vi "FDD Self TRAINING Polynomial FIT Ver07.vi"(4 "Remove Coefficient\nif makes < X% Change in SSE":dbl=1.0, 5 "DO Backward Elimination\nto REDUCE # Coefficients?":bool, 7 "No Header Labels?":bool, 8 "Select Polynomial Order":u16(ring) items=["1st ORDER", "2nd ORDER", "3rd Order"], 9 "Dependent Variable\nCOLUMN INDICES":i32[](array[numeric])=[5, 6, 8, 9, 12, 22, 39, 40, 46, 47, 48, 49, 54, 58, 64, 65, 69, 77, 81, 82, 87, 90, 92, 93, 105, 134, 135, 185, 188, 191, 192, 194, 206, 207, 208, 209, 210, 211, 219, 220, 222, 223, 225, 226, 227, 228, 229, 230, 231, 232, 233, 234, 237, 240, 241, 245, 246, 252, 254, 255, 256, 258, 260, 267, 268, 269], 10 "THREE Independent Variables\nCOLUMN INDICES":i32[](array[numeric])=[182, 83, 195]) -> (0 "# of Points (ROWS)":i32, 1 "Dependent VARIABLE(S) Numeric Data Array":dbl[][](array[numeric]), 2 "Independent VARIABLES, x1, x2, x3 -  Numeric Data Array":dbl[][](array[numeric]), 3 "Reduced Model(s) Coefficients with MSE, DOF(N-m), Student T-Value, and Model 95% CI (on Mean) in last four columns of the row":string[][](array[string]), 11 "RAW Data Array - STRING":string[][](array[string])=[["Hughie", "Dewey", "Louie", "Daffy", "Daisy"], ["1", "11", "4587", "4756", "12"], ["4", "55", "46", "5458", "45"], ["2", "22", "4789", "4445", "44"], ["7", "77", "258", "7595", "78"], ["9", "22", "1125", "147", "44545"], ["12", "33", "567", "233", "44"], ["32", "88", "413", "546", "895"], ["23", "65", "789", "7778", "458"], ["67", "99", "599", "6754", "478"], ["2111", "345", "678", "4399", "155"], ["199", "34", "555", "3987", "225"], ["37", "145", "258", "458", "3655"], ["876", "74", "635", "1258", "479"], ["45", "69", "158", "635", "258"], ["23", "125", "365", "489", "895"], ["11", "48", "428", "569", "965"], ["78", "79", "123", "45", "995"], ["65", "225", "754", "478", "788"], ["11", "48", "982", "569", "774"], ["97", "49", "4289", "483", "258"], ["38", "698", "1587", "147", "88"]])   [LabVIEW 2017]
uses:
  Control 1.ctl
  <vilib>/Analysis/6fits.llb/Curve Fitting Criteria.ctl
  <vilib>/Analysis/6fits.llb/General Linear Fit Algorithm.ctl
  <vilib>/Analysis/baseanly.llb/Mean (DBL).vi
  <vilib>/Utility/file.llb/Read Delimited Spreadsheet (string).vi
  <vilib>/Utility/file.llb/Write Delimited Spreadsheet (string).vi
  <vilib>/gmath/statdist.llb/st_Percentiles (scalar).vi
  <vilib>/Analysis/NI_AALPro.lvlib
  <vilib>/Analysis/NI_AALBase.lvlib
  <vilib>/gmath/NI_Gmath.lvlib
panel:
  out "Full Model # of Coef.":i32
  out "Current Input FILE":string
  out "STOPPED 2":bool
  out "STOPPED":bool
  out "General Linear FIT error out":errorcluster
  in  "Tab Control":T1(tab)
  in  "SAVE?":bool
  in  "Saved Coefficient File":path=path "C:/TEMP/Coef_JUNK_Goodman_SHORT_COOL_NFSS_ALL_161207.txt"
  in  "Process\nData ??":bool
  in  "Input File":path=path "C:/Vance/FDD Split System Project/FDD_LOW-HIGH_EfficiencyHP_Testing/Goodman 14SEER Single-Speed HP LOW EFF UNIT TESTS 2015-16/SHORT LINESET DATA/Test DATA/BINS_Goodman_SHORT_COOL_NFSS_ALL_161207.txt"
  out "Save Coeff error out":errorcluster
  out "RAW Data COLUMN HEADER LABELS":string[](array[string])
  in  "Array of Calculated Variables (stuck in columns at end of Data Array String)":T3(array[cluster])=[{"Test Function"=7, "USE CONST."=FALSE, "CONSTANT"=1.0, "DATA COLUMNS"=[56.0, 60.0], "NEW HEADER LABEL"="ODAir_Exit_TempF"}, {"Test Function"=8, "USE CONST."=FALSE, "CONSTANT"=1.0, "DATA COLUMNS"=[266.0, 195.0], "NEW HEADER LABEL"="ODAir_DT(F)"}, {"Test Function"=8, "USE CONST."=FALSE, "CONSTANT"=1.0, "DATA COLUMNS"=[82.0, 105.0], "NEW HEADER LABEL"="LiqLine_DP(psid)"}]
  out "RAW & Calculated Data COLUMN HEADER LABELS":string[](array[string])
  in  "PAUSE to Select Independent \nand Dependent Data COLUMNS":bool
  out "RAW & CALCULATED Data Array - STRING":string[][](array[string])=[["Hughie", "Dewey", "Louie", "Daffy", "Daisy"], ["1", "11", "4587", "4756", "12"], ["4", "55", "46", "5458", "45"], ["2", "22", "4789", "4445", "44"], ["7", "77", "258", "7595", "78"], ["9", "22", "1125", "147", "44545"], ["12", "33", "567", "233", "44"], ["32", "88", "413", "546", "895"], ["23", "65", "789", "7778", "458"], ["67", "99", "599", "6754", "478"], ["2111", "345", "678", "4399", "155"], ["199", "34", "555", "3987", "225"], ["37", "145", "258", "458", "3655"], ["876", "74", "635", "1258", "479"], ["45", "69", "158", "635", "258"], ["23", "125", "365", "489", "895"], ["11", "48", "428", "569", "965"], ["78", "79", "123", "45", "995"], ["65", "225", "754", "478", "788"], ["11", "48", "982", "569", "774"], ["97", "49", "4289", "483", "258"], ["38", "698", "1587", "147", "88"]]
  out "Selected CASE":i32
  out "H Matrix":dbl[][](array[numeric])
  out "FULL Dataset Correlation Coefficients  and MSE in last column of the row (a0, a1, a2, ......., MSE)":dbl[][](array[numeric]) format="%_8e"
  in  "Outlier IQR Multiplier (k)":dbl=2.2
  out "Residuals for all Dependent Variables (Value Minus Fit Value)":dbl[][](array[numeric]) format="%_8e"
  out "STATS Columns for each Dependent Variable's Residuals":dbl[][](array[numeric]) format="%_4p"
  out "% of Data = OUTLIER":dbl format="%_3f"
  out "# OUTLIERS":i32
  out "# Datapoints in File":i32
  out "Residual's Variable NAME 2":string
  out "Line Numbers w/ OUTLIERS":bool[](array[boolean])
  out "Outlier Identified (Row is Line #, Column is Variable #)":bool[][](array[boolean])
  out "Column w/ OUTLIER??":cluster{"Variable LABEL NAME":string, bool}[](array[cluster])
  out "Residual's Histogram Graph":T4(graph)
  in  "Histogram\nSelected COL":i32
  out "Residual Value vs Line # XY Graph":cluster{"Y":dbl[], "Y":dbl[]}[](graph)
  out "Skewness":dbl
  out "Kurtosis":dbl
  out "Residual's Variable NAME":string
  out "STATISTICS - Array 3":T5(array[cluster])
  out "STATISTICS - Array 2":T5(array[cluster])
  out "STATISTICS - Array":T5(array[cluster])
  out "TOSS OUT Coefficients indicated by RED LED's":bool[][](array[boolean])
  out "Reduced Model's H Matrix":dbl[][](array[numeric])
  out "F-Test----SSE Reduced Model(s) Divided by SSE Full Model = SSE Ratio":dbl[][](array[numeric]) format="%.3p"
  out "SSE Full Model(s)":dbl[](array[numeric])
  out "SSE Ratio Must Be < THIS \nto Throw Out the Coeff.":dbl format="%#_6p"
  out "ERROR CODE":i32
  out "Dependent \nVariable INDEX":i32
  in  "10 sec Pause\nSTEP to Debug?":bool
  out "Fitted Coefficients MATRIX \nAssociated with H-Matrix w/ MSE at END":dbl[](array[numeric])
  out "Dependent Variable MATRIX \nAssociated with H-Matrix":dbl[](array[numeric])
  out "H-Matrix AFTER ZERO Value COLS ADDED":dbl[][](array[numeric]) format="%_9e"
  out "Coefficients with MSE in last Column-NUMERIC ARRAY":dbl[][](array[numeric]) format="%_9e"
  out "Reduced Model \n# of Coefficients":i32
  out "#COLS":i32
  # "Multivariate Polynomial FIT with 3 Independent Variables"
  # "y = a0*y0 + a1*y1 + .....+ai*yi  \nwhere i =0 to 19.\ny0=1;\ny1=x1;\ny2=x2;              1st Order\ny3=x3;\n--------------\ny4=x1*x2;\ny5=x1*x3;\ny6=x2*x3;\ny7=x1**2;        2nd Order\ny8=x2**2;\ny9=x3**2;\n----------------\ny10=x1*x2*x3;\ny11=x1*x2**2;\ny12=x1*x3**2;\ny13=x2*x3**2;\ny14=x1**2*x2;  3rd Order\ny15=x1**2*x3;\ny16=x2**2*x3;\ny17=x1**3;\ny18=x2**3;\ny19=x3**3;"
  # "Needs to be a Tab Delimited Text file \nwith data in columns."
  # "Max\nMin\nMedian\nQuartile 1 (25%)\nQuartile 3 (75%)\nInterQuartileRange (3-1)\nOutlier LowerBound\nOutlier UpperBound"
  # "LowerBound = Q1 - k * IQR\nUpperBound = Q3 + k * IQR"
  # "Assumes Residuals are normally distributed about zero."
  # "A negative value of skewness indicates \nthat the left side of the probability density \nfunction is longer than the right side. A \npositive value of skewness indicates that \nthe right side of the probability density \nfunction is longer than the left side."
  # "A normal distribution has a kurtosis value \nof 3. A kurtosis value of less than 3 indicates \na flatter distribution than normal. A kurtosis \nvalue of greater than 3 indicates a sharper \ndistribution than normal."
  # "For Example:\n(0,0) is the SSE Ratio after removing a0 from Model 0\n(1,2) is the SSE Ratio after removing a2 from Model 2"
  # "If you have only one Independent Variable,\nthen you will have only ONE row of SSE ratio."
  # "Each COL is replaced by 0's in sequence to remove the coefficent from the fit.  \nFinal ARRAY will show all 0's in the last COL."
  # "Degrees of Freedom\n= DOF = #Points-#Coef = N-m"
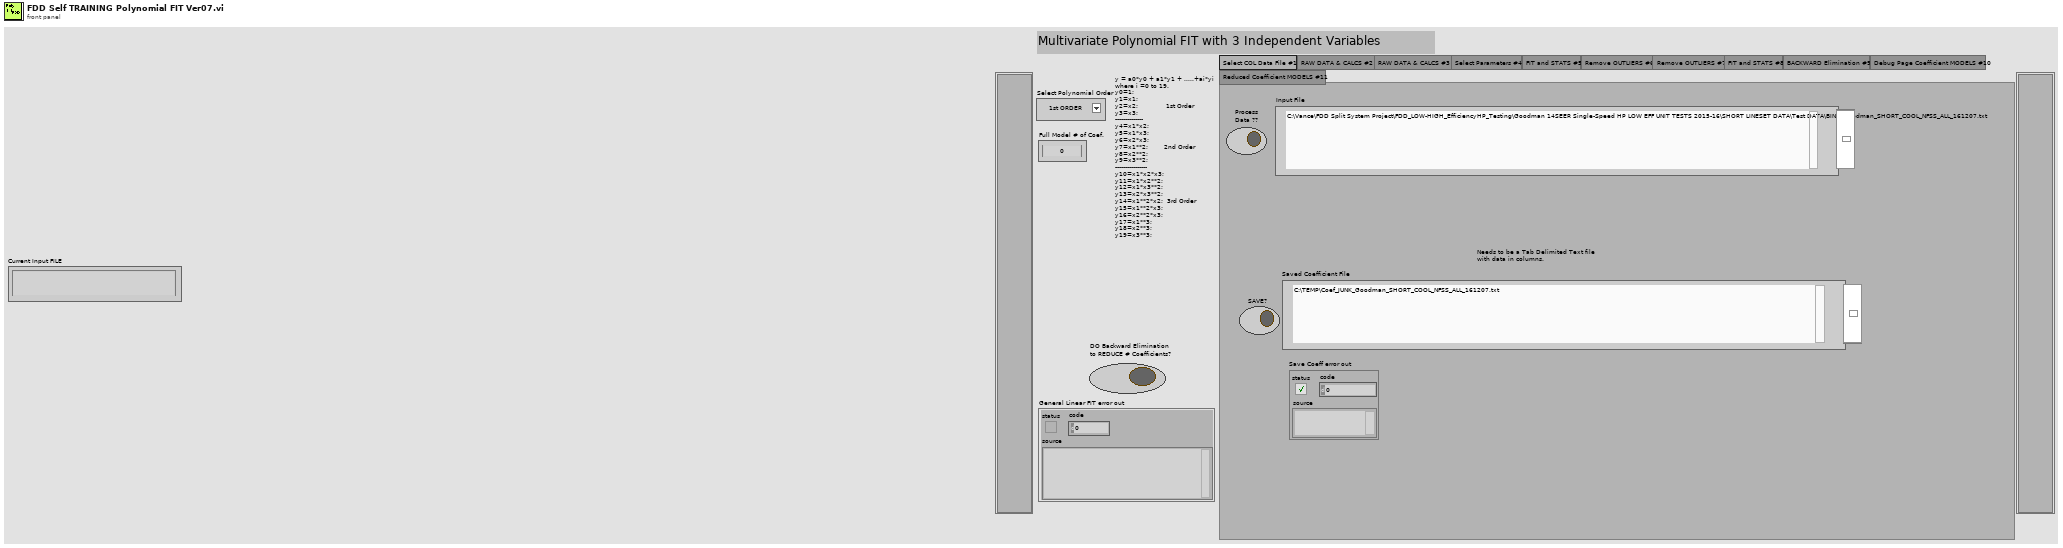
[diagram p1: front panel]
types:
  T1 = enum32{"Select COL Data File #1", "RAW DATA & CALCS #2", "RAW DATA & CALCS #3", "Select Parameters #4", "FIT and STATS #5", "Remove OUTLIERS #6", "Remove OUTLIERS #7", "FIT and STATS #8", "BACKWARD Elimination #9", "Debug Page Coefficient MODELS #10", "Reduced Coefficient MODELS #11"}
  T2 = typedef "Control 1.ctl" = i32
  T3 = cluster{"Test Function":T2, "USE CONST.":bool, "CONSTANT":dbl, "DATA COLUMNS":dbl[], "NEW HEADER LABEL":string}[]
  T4 = cluster{"X Values":dbl[], "Histogram: h(x)":i32[]}
  T5 = cluster{"Header":string, "Mean":dbl, "Std. Dev":dbl, "MAX":dbl, "MIN":dbl, "Range":dbl}[]
  T6 = cluster{"String":string, "mean":dbl, "standard deviation":dbl, dbl, dbl, dbl}
  T7 = typedef "NI_AALPro.lvlib/General Linear Fit Algorithm.ctl" = u16
  T8 = typedef "NI_AALPro.lvlib/Curve Fitting Criteria.ctl" = u16
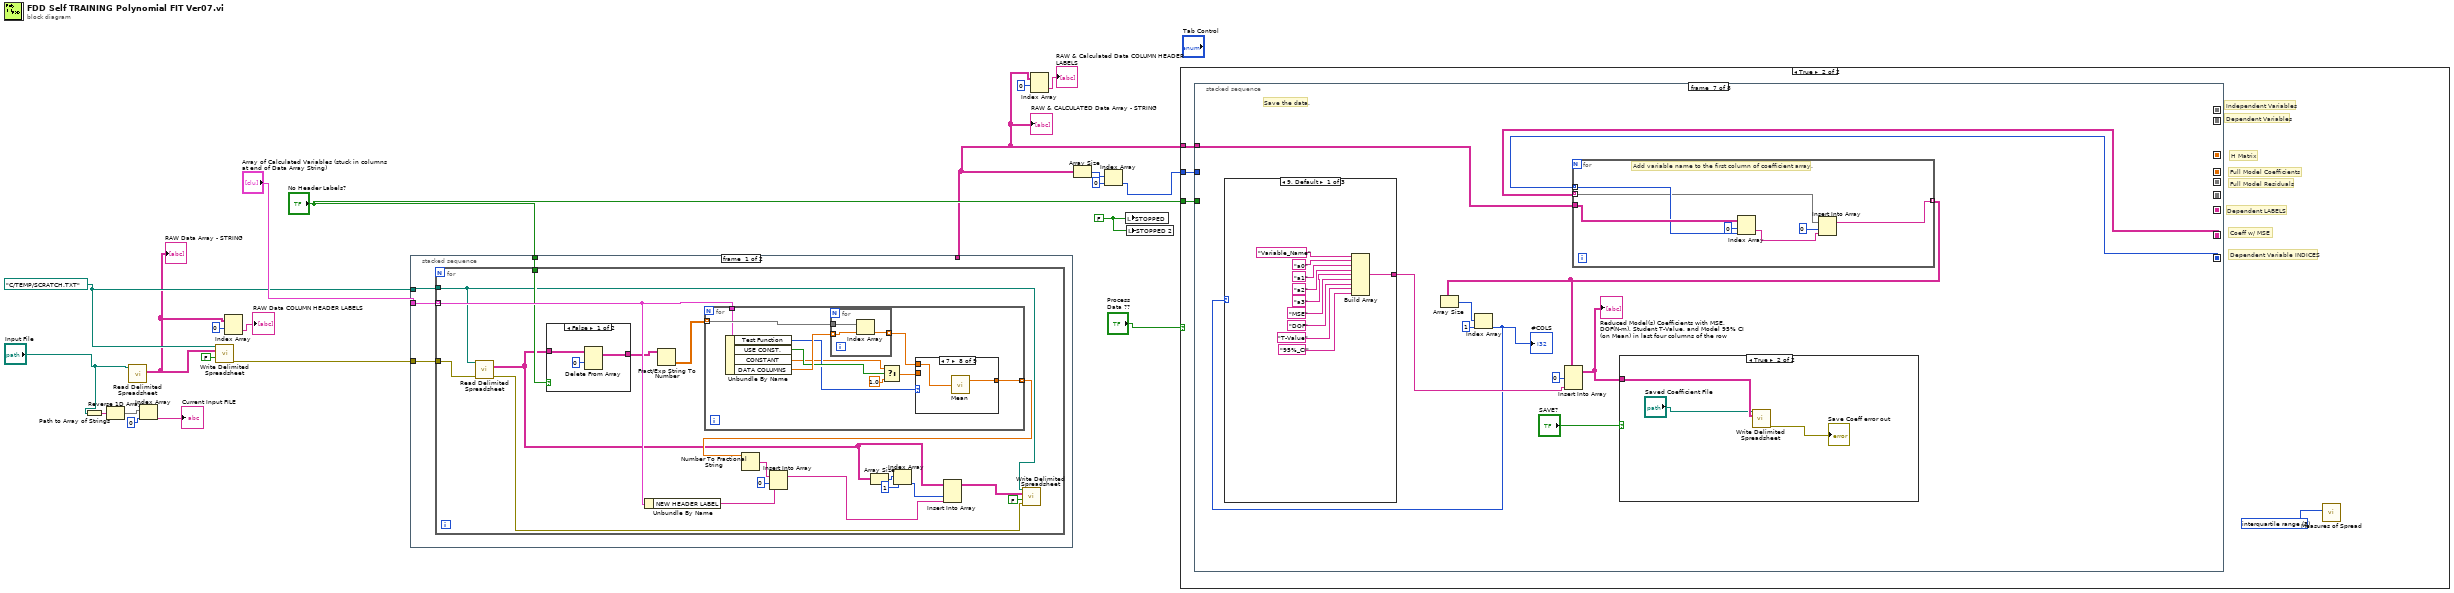
[diagram p0: block diagram]
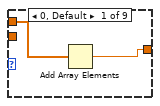
[diagram p3: hidden frame]
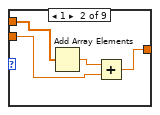
[diagram p4: hidden frame]
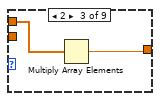
[diagram p5: hidden frame]
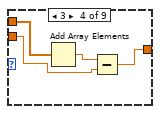
[diagram p6: hidden frame]
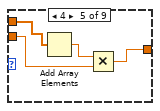
[diagram p7: hidden frame]
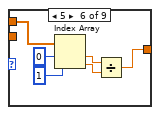
[diagram p8: hidden frame]
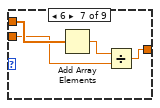
[diagram p9: hidden frame]
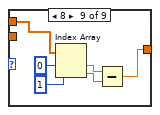
[diagram p10: hidden frame]
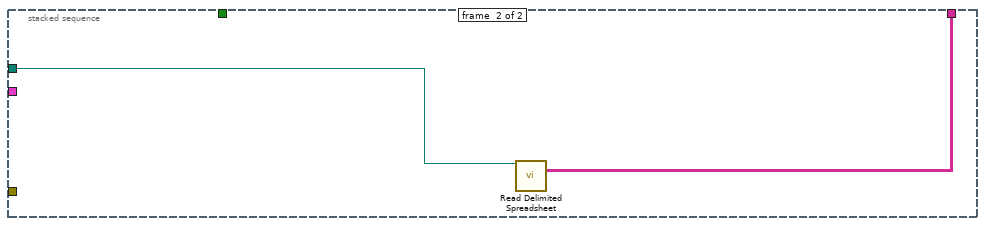
[diagram p11: hidden frame]
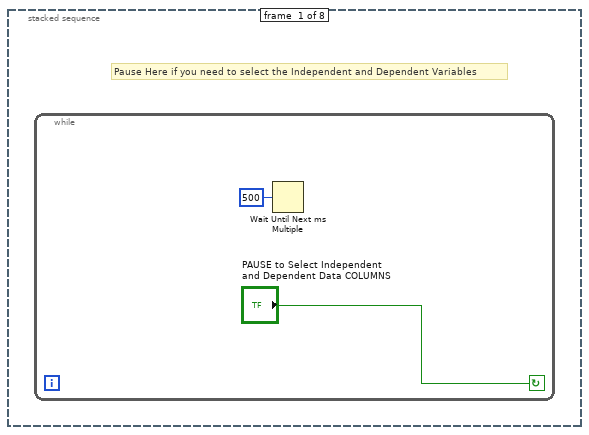
[diagram p13: hidden frame]
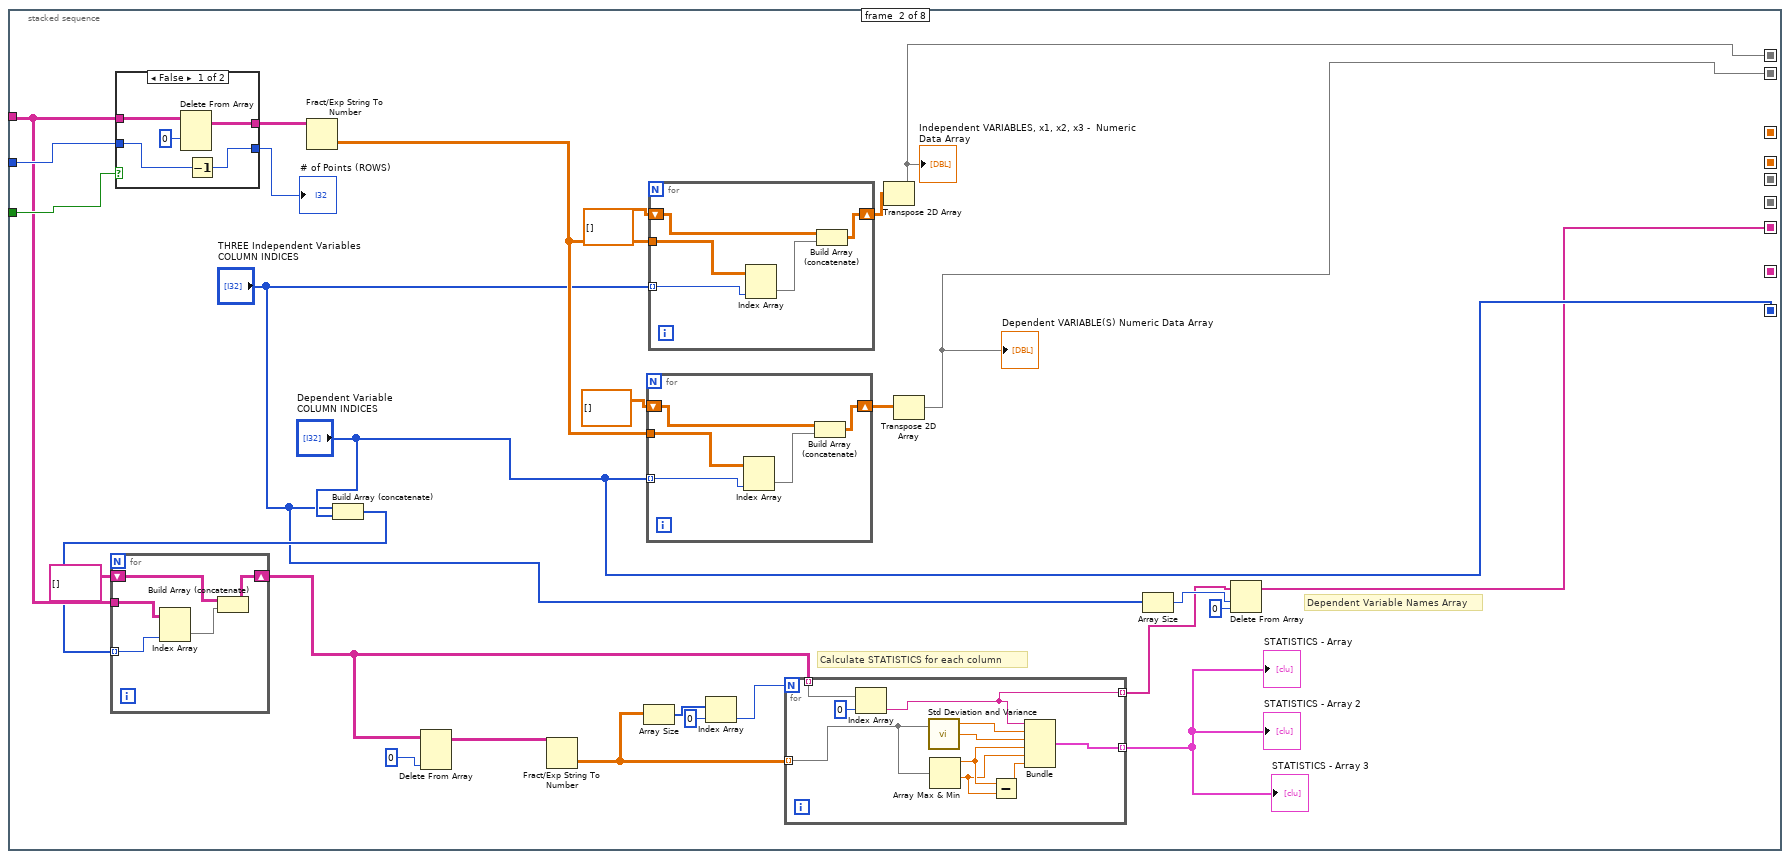
[diagram p14: hidden frame]
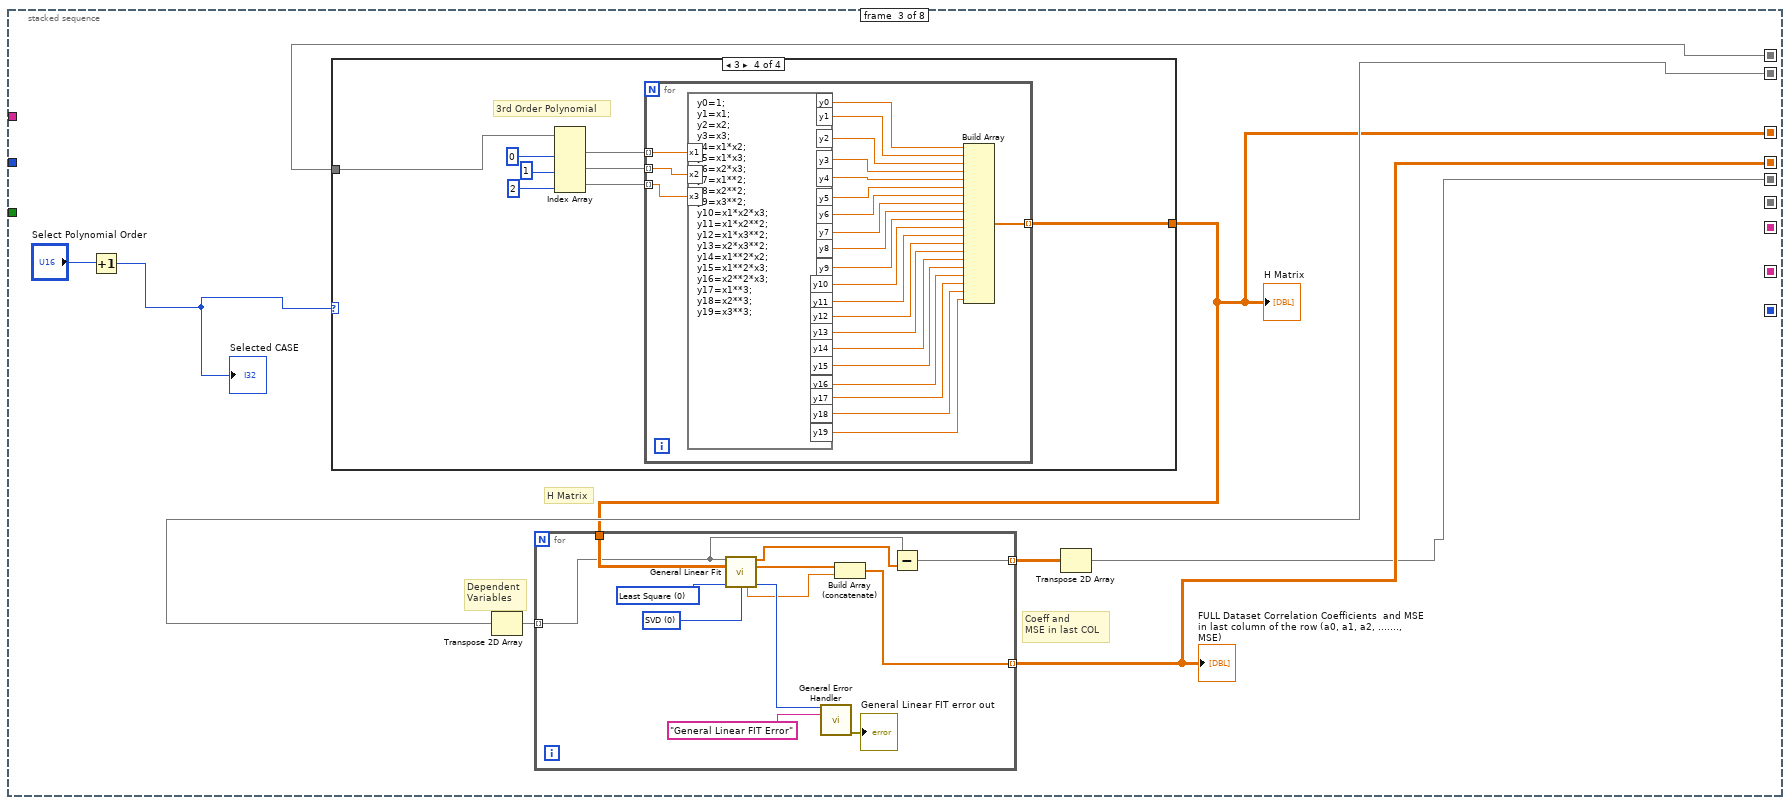
[diagram p16: hidden frame]
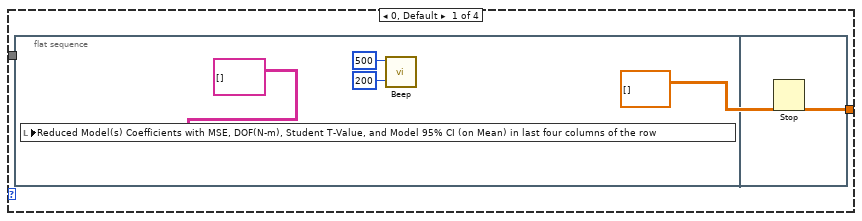
[diagram p17: hidden frame]
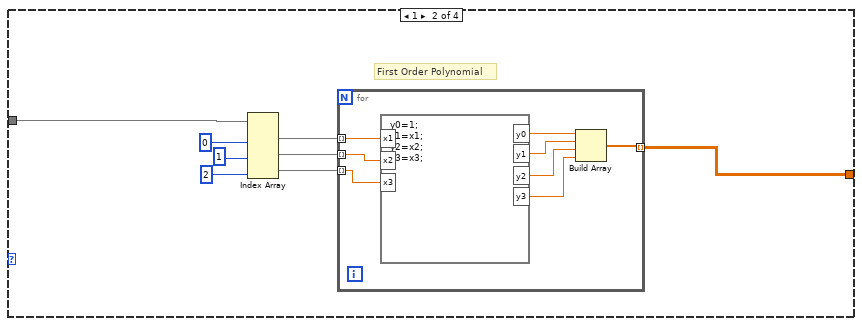
[diagram p18: hidden frame]
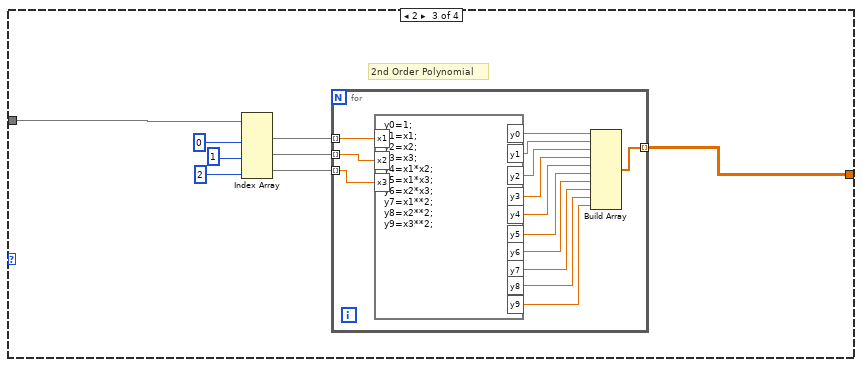
[diagram p19: hidden frame]
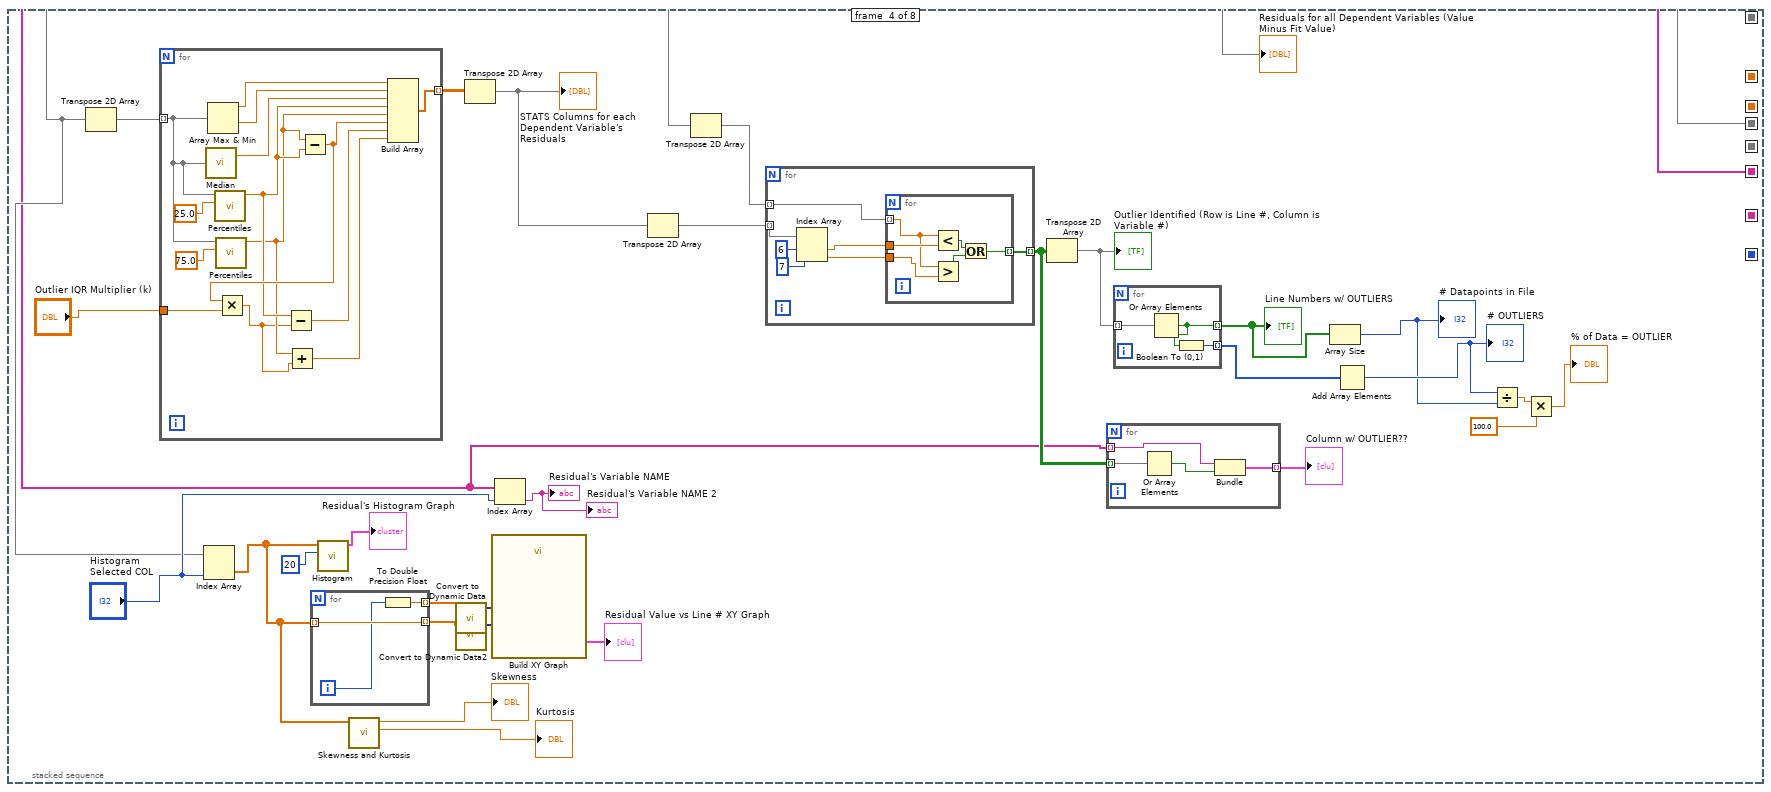
[diagram p20: hidden frame]
diagram:
  w7 = path "C:/TEMP/SCRATCH.TXT" ("file path (dialog if empty)")
  w18 = FALSE ("STOPPED")
  n1 = Path to Array of Strings(0:"Input File") -> (2:w14:string[])  [unwired: 1 out]
  n2 = Reverse 1D Array(array=w14) -> (reversed array=w13:string[])
  n3 = call-poly <vilib>:"Read Delimited Spreadsheet.vi"("file path (dialog if empty)"="Input File") -> ("all rows"=w1:string[][])  [unwired: 9 in, 5 out]
  "RAW Data Array - STRING" <- w1
  n4 = Index Array(array=w13, index=0) -> (element=→"Current Input FILE":string)
  n5 = call-poly <vilib>:"Write Delimited Spreadsheet.vi"("file path (dialog if empty)"=w7, "2D data"=w1, "append to file? (new file:F)"=FALSE ("append to file? (F)")) -> ("error out"=w8:errorcluster)  [unwired: 11 in, 1 out]
  n6 = Index Array(array=w1, index (row)=0) -> (element=→"RAW Data COLUMN HEADER LABELS":string[])  [unwired: 1 in]
  n7 = stacked-sequence {
    tunnel: "Array of Calculated Variables (stuck in columns at end of Data Array String)" -> [w25 _]
    tunnel: "No Header Labels?" -> [w24 _]
    tunnel: w8 -> [w23 _]
    tunnel: w7 -> [w22 w96]
    tunnel: [_ w95] -> w5
    frame #0 {
      n8 = for {
        tunnel: w25 -> [w39] mode=indexing
        tunnel: w24 -> [w37]
        tunnel: w22 -> [w29]
        tunnel: w23 -> [w28]
        n9 = call-poly <vilib>:"Read Delimited Spreadsheet.vi"("file path (dialog if empty)"=w29, "error in (no error)"=w28) -> ("all rows"=w30:string[][], "error out"=w27:errorcluster)  [unwired: 8 in, 4 out]
        n10 = case shown="False" w37 {
          tunnel: w30 -> [w46 w47]
          tunnel: [w44 w47] -> w38
          frame False {
            n11 = Delete From Array(array=w46, index (row)=0) -> (array with subset deleted=w44:string[][])  [unwired: 2 in, 1 out]
          }
          frame True {
          }
        }
        n12 = Unbundle By Name(w39) -> ("NEW HEADER LABEL"=w43:string)
        n13 = Fract/Exp String To Number(string=w38) -> (number=w36:dbl[][])  [unwired: 3 in, 1 out]
        n14 = for {
          tunnel: w36 -> [w57] mode=indexing
          tunnel: w39 -> [w55]
          tunnel: [w48] -> w41 mode=indexing
          n15 = Unbundle By Name(w55) -> ("Test Function"=w52:T2, "USE CONST."=w53:bool, "CONSTANT"=w51:dbl, "DATA COLUMNS"=w54:dbl[])
          n16 = for {
            tunnel: w57 -> [w60]
            tunnel: w54 -> [w59] mode=indexing
            tunnel: [w58] -> w49 mode=indexing
            n17 = Index Array(array=w60, index=w59) -> (element=w58:dbl)
          }
          n18 = Select(t=w51, s=w53, f=1.0) -> (s? t:f=w56:dbl)
          n19 = case shown="7" w52 {
            tunnel: w56 -> [_ w64 _ w70 w74 _ w84 _ _]
            tunnel: [w61 w63 w67 w69 w73 w77 w83 w87 w89] -> w48
            tunnel: w49 -> [w62 w66 w68 w72 w75 w82 w85 w88 w90]
            frame 0, Default {
              n20 = Add Array Elements(numeric array=w62) -> (sum=w61:dbl)
            }
            frame 1 {
              n21 = Add Array Elements(numeric array=w66) -> (sum=w65:dbl)
              n22 = Add(x=w65, y=w64) -> (x+y=w63:dbl)
            }
            frame 2 {
              n23 = Multiply Array Elements(1:w68) -> (0:w67:dbl)
            }
            frame 3 {
              n24 = Add Array Elements(numeric array=w72) -> (sum=w71:dbl)
              n25 = Subtract(x=w71, y=w70) -> (x-y=w69:dbl)
            }
            frame 4 {
              n26 = Add Array Elements(numeric array=w75) -> (sum=w76:dbl)
              n27 = Multiply(x=w76, y=w74) -> (x*y=w73:dbl)
            }
            frame 5 {
              n28 = Index Array(array=w82, index #1=0 ("index"), index #2=1 ("index")) -> (element #1=w79:dbl, element #2=w78:dbl)
              n29 = Divide(x=w79, y=w78) -> (x/y=w77:dbl)
            }
            frame 6 {
              n30 = Add Array Elements(numeric array=w85) -> (sum=w86:dbl)
              n31 = Divide(x=w86, y=w84) -> (x/y=w83:dbl)
            }
            frame 7 {
              n32 = call-poly <vilib>:"Mean.vi"("X"=w88) -> ("mean"=w87:dbl)  [unwired: 1 out]
            }
            frame 8 {
              n33 = Index Array(array=w90, index #1=0 ("index"), index #2=1 ("index")) -> (element #1=w92:dbl, element #2=w91:dbl)
              n34 = Subtract(x=w92, y=w91) -> (x-y=w89:dbl)
            }
          }
        }
        n35 = Number To Fractional String(number=w41) -> (F-format string=w40:string[])  [unwired: 3 in]
        n36 = Insert Into Array(array=w40, index=0, new element=w43) -> (w26:string[])
        n37 = Array Size(array=w30) -> (size(s)=w33:i32[])
        n38 = Index Array(array=w33, index=1) -> (element=w31:i32)
        n39 = Insert Into Array "Insert Into Array"(array=w30, index (col)=w31, new element=w26) -> (w34:string[][])  [unwired: 1 in]
        n40 = call-poly <vilib>:"Write Delimited Spreadsheet.vi"("file path (dialog if empty)"=w29, "2D data"=w34, "append to file? (new file:F)"=FALSE ("append to file? (F)"), "error in (no error)"=w27) -> ()  [unwired: 10 in, 2 out]
      }
    }
    frame #1 {
      n41 = call-poly <vilib>:"Read Delimited Spreadsheet.vi"("file path (dialog if empty)"=w96) -> ("all rows"=w95:string[][])  [unwired: 9 in, 5 out]
    }
  }
  "RAW & CALCULATED Data Array - STRING" <- w5
  n42 = Index Array(array=w5, index (row)=0) -> (element=→"RAW & Calculated Data COLUMN HEADER LABELS":string[])  [unwired: 1 in]
  n43 = Array Size(array=w5) -> (size(s)=w21:i32[])
  n44 = Index Array(array=w21, index=0) -> (element=w19:i32)
  n45 = local write "STOPPED"(w18) -> ()
  n46 = local write "STOPPED 2"(w18) -> ()
  n47 = case shown="True" "Process\nData ??" {
    tunnel: w19 -> [_ w100]
    tunnel: w5 -> [_ w99]
    tunnel: "No Header Labels?" -> [_ w98]
    frame False {
    }
    frame True {
      w97 = 3 items=["standard deviation", "range", "mean absolute deviation", "interquartile range"] ("type")
      # "Dependent LABELS"
      # "Full Model Residuals"
      # "Coeff w/ MSE"
      # "Dependent Variable INDICES"
      # "H Matrix"
      # "Full Model Coefficients"
      # "Independent Variables"
      # "Dependent Variables"
      n48 = stacked-sequence {
        seq-local: [_ w124 _ _ _ _ _ _] -> [_ _ w171 _ _ _ _ _]
        seq-local: [_ w123 _ _ _ _ _ _] -> [_ _ w170 _ w343 w394 _ _]
        seq-local: [_ _ w168 _ _ _ _ _] -> [_ _ _ _ w329 w390 _ _]
        seq-local: [_ _ w167 _ _ _ _ _] -> [_ _ _ _ w341 w392 _ _]
        seq-local: [_ _ _ _ w332 _ _ _] -> [_ _ _ _ _ w393 _ _]
        seq-local: [_ _ _ _ _ w389 _ _] -> [_ _ _ _ _ _ w479 _]
        seq-local: [_ "Dependent Variable\nCOLUMN INDICES" _ _ _ _ _ _] -> [_ _ _ _ _ _ w481 _]
        seq-local: [_ _ w163 _ _ _ _ _] -> [_ _ _ w272 _ _ _ _]
        seq-local: [_ w103 _ _ _ _ _ _] -> [_ _ _ w267 _ _ _ _]
        tunnel: w99 -> [_ w114 _ _ _ _ w480 _]
        tunnel: w100 -> [_ w122 _ _ w344 _ _ _]
        tunnel: w98 -> [_ w120 _ _ _ _ _ _]
        frame #0 {
          # "Pause Here if you need to select the Independent and Dependent Variables"
          n49 = while {
            stop <- "PAUSE to Select Independent \nand Dependent Data COLUMNS" continue-if-true
            n50 = Wait Until Next ms Multiple(millisecond multiple=u32 500) -> ()  [unwired: 1 out]
          }
        }
        frame #1 {
          # "Dependent Variable Names Array"
          # "Calculate STATISTICS for each column"
          n51 = case shown="False" w120 {
            tunnel: w114 -> [w160 w162]
            tunnel: [w158 w162] -> w130
            tunnel: w122 -> [w157 w161]
            tunnel: [w156 w161] -> w121
            frame False {
              n52 = Delete From Array(array=w160, index (row)=0) -> (array with subset deleted=w158:string[][])  [unwired: 2 in, 1 out]
              n53 = Decrement(x=w157) -> (x-1=w156:i32)
            }
            frame True {
            }
          }
          "# of Points (ROWS)" <- w121
          n54 = Fract/Exp String To Number(string=w130) -> (number=w127:dbl[][])  [unwired: 3 in, 1 out]
          n55 = Build Array (concatenate)("THREE Independent Variables\nCOLUMN INDICES", "Dependent Variable\nCOLUMN INDICES") -> (w113:i32[])
          n56 = for {
            tunnel: w114 -> [w135]
            tunnel: w113 -> [w134] mode=indexing
            shift-right: [w132] -> w110
            shift-left: string[][] [] -> [w131]
            n57 = Index Array(array=w135, index (col)=w134) -> (element=w133:string[])  [unwired: 1 in]
            n58 = Build Array (concatenate)(w131, w133) -> (w132:string[][])
          }
          n59 = Delete From Array "Delete From Array"(array=w110, index (col)=0 ("index (row)")) -> (array with subset deleted=w119:string[][])  [unwired: 2 in, 1 out]
          n60 = Fract/Exp String To Number(string=w119) -> (number=w109:dbl[][])  [unwired: 3 in, 1 out]
          n61 = Array Size(array=w109) -> (size(s)=w118:i32[])
          n62 = for {
            tunnel: w127 -> [w150]
            tunnel: "Dependent Variable\nCOLUMN INDICES" -> [w149] mode=indexing
            shift-right: [w147] -> w125
            shift-left: dbl[][] [] -> [w146]
            n63 = Index Array(array=w150, index (col)=w149) -> (element=w148:dbl[])  [unwired: 1 in]
            n64 = Build Array (concatenate)(w146, w148) -> (w147:dbl[][])
          }
          n65 = for {
            tunnel: w127 -> [w155]
            tunnel: "THREE Independent Variables\nCOLUMN INDICES" -> [w154] mode=indexing
            shift-right: [w152] -> w126
            shift-left: dbl[][] [] -> [w151]
            n66 = Index Array(array=w155, index (col)=w154) -> (element=w153:dbl[])  [unwired: 1 in]
            n67 = Build Array (concatenate)(w151, w153) -> (w152:dbl[][])
          }
          n68 = Index Array(array=w118, index=0) -> (element=w116:i32)
          n69 = for {
            N: w116 -> [_]
            tunnel: w109 -> [w143] mode=indexing
            tunnel: [w139] -> w111 mode=indexing
            tunnel: w110 -> [w138] mode=indexing
            tunnel: [w136] -> w104 mode=indexing
            n70 = Index Array(array=w138, index=0) -> (element=w136:string)
            n71 = call <vilib>:"Std Deviation and Variance.vi"("X"=w143) -> ("mean"=w145:dbl, "standard deviation"=w144:dbl)  [unwired: 1 in, 1 out]
            n72 = Array Max & Min(array=w143) -> (max value=w142:dbl, min value=w141:dbl)  [unwired: 2 out]
            n73 = Subtract(x=w142, y=w141) -> (x-y=w140:dbl)
            n74 = Bundle("String"=w136, "mean"=w145, "standard deviation"=w144, w142, w141, w140) -> (w139:T6)  [unwired: 1 in]
          }
          "STATISTICS - Array" <- w111
          "STATISTICS - Array 3" <- w111
          "STATISTICS - Array 2" <- w111
          n75 = Transpose 2D Array(2D array=w126) -> (transposed array=w124:dbl[][])
          "Independent VARIABLES, x1, x2, x3 -  Numeric Data Array" <- w124
          n76 = Transpose 2D Array(2D array=w125) -> (transposed array=w123:dbl[][])
          "Dependent VARIABLE(S) Numeric Data Array" <- w123
          n77 = Array Size(array="THREE Independent Variables\nCOLUMN INDICES") -> (size(s)=w105:i32)
          n78 = Delete From Array(array=w104, length=w105, index=0) -> (array with subset deleted=w103:string[])  [unwired: 1 out]
        }
        frame #2 {
          # "Coeff and\nMSE in last COL"
          # "H Matrix"
          # "Dependent\nVariables"
          n79 = Increment(x="Select Polynomial Order") -> (x+1=w165:u16)
          "Selected CASE" <- w165
          n80 = case shown="3" w165 {
            tunnel: w171 -> [_ w195 w205 w227]
            tunnel: [dbl[][] [] w188 w204 w226] -> w167
            frame 0, Default {
              n81 = flat-sequence {
                frame #0 {
                  n82 = local write "Reduced Model(s) Coefficients with MSE, DOF(N-m), Student T-Value, and Model 95% CI (on Mean) in last four columns of the row"(string[][] []) -> ()
                  n83 = call <vilib>:"Beep.vi"("duration (msec)"=u32 200, "frequency (Hz)"=u32 500) -> ()  [unwired: 10 in]
                }
                frame #1 {
                  n84 = Stop() -> ()  [unwired: 1 in]
                }
              }
            }
            frame 1 {
              # "First Order Polynomial"
              n85 = Index Array(array=w195, index (col) #1=0 ("index"), index (col) #2=1 ("index"), index (col) #3=2 ("index")) -> (element #1=w191:dbl[], element #2=w190:dbl[], element #3=w189:dbl[])  [unwired: 3 in]
              n86 = for {
                tunnel: w191 -> [w203] mode=indexing
                tunnel: w190 -> [w202] mode=indexing
                tunnel: w189 -> [w201] mode=indexing
                tunnel: [w196] -> w188 mode=indexing
                n87 = formula code="y0=1;\ny1=x1;\ny2=x2;\ny3=x3;"("x1"=w203, "x2"=w202, "x3"=w201) -> ("y0"=w200:dbl, "y1"=w199:dbl, "y2"=w198:dbl, "y3"=w197:dbl)
                n88 = Build Array(w200, w199, w198, w197) -> (w196:dbl[])
              }
            }
            frame 2 {
              # "2nd Order Polynomial"
              n89 = Index Array(array=w205, index (col) #1=0 ("index"), index (col) #2=1 ("index"), index (col) #3=2 ("index")) -> (element #1=w208:dbl[], element #2=w207:dbl[], element #3=w206:dbl[])  [unwired: 3 in]
              n90 = for {
                tunnel: w208 -> [w225] mode=indexing
                tunnel: w207 -> [w224] mode=indexing
                tunnel: w206 -> [w223] mode=indexing
                tunnel: [w218] -> w204 mode=indexing
                n91 = formula code="y0=1;\ny1=x1;\ny2=x2;\ny3=x3;\ny4=x1*x2;\ny5=x1*x3;\ny6=x2*x3;\ny7=x1**2;\ny8=x2**2;\ny9=x3**2;"("x1"=w225, "x2"=w224, "x3"=w223) -> ("y0"=w222:dbl, "y1"=w221:dbl, "y2"=w220:dbl, "y3"=w219:dbl, "y4"=w217:dbl, "y5"=w216:dbl, "y6"=w215:dbl, "y7"=w214:dbl, "y8"=w213:dbl, "y9"=w212:dbl)
                n92 = Build Array(w222, w221, w220, w219, w217, w216, w215, w214, w213, w212) -> (w218:dbl[])
              }
            }
            frame 3 {
              # "3rd Order Polynomial"
              n93 = Index Array(array=w227, index (col) #1=0 ("index"), index (col) #2=1 ("index"), index (col) #3=2 ("index")) -> (element #1=w230:dbl[], element #2=w229:dbl[], element #3=w228:dbl[])  [unwired: 3 in]
              n94 = for {
                tunnel: w230 -> [w257] mode=indexing
                tunnel: w229 -> [w256] mode=indexing
                tunnel: w228 -> [w255] mode=indexing
                tunnel: [w250] -> w226 mode=indexing
                n95 = formula code="y0=1;\ny1=x1;\ny2=x2;\ny3=x3;\ny4=x1*x2;\ny5=x1*x3;\ny6=x2*x3;\ny7=x1**2;\ny8=x2**2;\ny9=x3**2;\ny10=x1*x2*x3;\ny11=x1*x2**2;\ny12=x1*x3**2;\ny13=x2*x3**2;\ny14=x1**2*x2;\ny15=x1**2*x3;\ny16=x2**2*x3;\ny17=x1**3;\ny18=x2**3;\ny19=x3**3;"("x1"=w257, "x2"=w256, "x3"=w255) -> ("y0"=w254:dbl, "y1"=w253:dbl, "y2"=w252:dbl, "y3"=w251:dbl, "y4"=w249:dbl, "y5"=w248:dbl, "y6"=w247:dbl, "y7"=w246:dbl, "y8"=w245:dbl, "y9"=w244:dbl, "y10"=w243:dbl, "y11"=w242:dbl, "y12"=w241:dbl, "y13"=w240:dbl, "y14"=w239:dbl, "y15"=w238:dbl, "y16"=w237:dbl, "y17"=w236:dbl, "y18"=w235:dbl, "y19"=w234:dbl)
                n96 = Build Array(w254, w253, w252, w251, w249, w248, w247, w246, w245, w244, w243, w242, w241, w240, w239, w238, w237, w236, w235, w234) -> (w250:dbl[])
              }
            }
          }
          "H Matrix" <- w167
          n97 = Transpose 2D Array(2D array=w170) -> (transposed array=w169:dbl[][])
          n98 = for {
            tunnel: w169 -> [w174] mode=indexing
            tunnel: w167 -> [w183]
            tunnel: [w177] -> w168 mode=indexing
            tunnel: [w172] -> w164 mode=indexing
            w175 = T7 0 items=["SVD", "Givens", "Givens2", "Householder", "LU Decomposition", "Cholesky", "SVD for Rank Deficient H"] ("algorithm")
            w182 = T8 0 items=["Least Square", "Least Absolute Residual", "Bisquare"] ("method")
            n99 = call <vilib>:"General Linear Fit.vi"("Y"=w174, "H"=w183, "method"=w182, "algorithm"=w175) -> ("Best Fit"=w173:dbl[], "Coefficients"=w176:dbl[], "residue"=w178:dbl, "error"=w181:i32)  [unwired: 6 in, 2 out]
            n100 = call <vilib>:"General Error Handler.vi"("[error code] (0)"=w181, "[error source] (\" \")"="General Linear FIT Error" ("[error source] (\" \")")) -> ("error out"=→"General Linear FIT error out":errorcluster)  [unwired: 9 in, 4 out]
            n101 = Build Array (concatenate)(w176, w178) -> (w177:dbl[])
            n102 = Subtract(x=w174, y=w173) -> (x-y=w172:dbl[])
          }
          "FULL Dataset Correlation Coefficients  and MSE in last column of the row (a0, a1, a2, ......., MSE)" <- w168
          n103 = Transpose 2D Array(2D array=w164) -> (transposed array=w163:dbl[][])
        }
        frame #3 {
          n104 = Transpose 2D Array(2D array=w272) -> (transposed array=w285:dbl[][])
          n105 = for {
            tunnel: w285 -> [w318] mode=indexing
            tunnel: [w322] -> w287 mode=indexing
            tunnel: "Outlier IQR Multiplier (k)" -> [w316]
            n106 = call <vilib>:"Median.vi"("X"=w318) -> ("median"=w321:dbl)  [unwired: 1 out]
            n107 = Array Max & Min(array=w318) -> (max value=w324:dbl, min value=w323:dbl)  [unwired: 2 out]
            n108 = call-poly <vilib>:"Percentiles.vi"("p"=25.0, "x array"=w318) -> ("percentile"=w315:dbl)  [unwired: 8 in, 1 out]
            n109 = call-poly <vilib>:"Percentiles.vi"("p"=75.0, "x array"=w318) -> ("percentile"=w314:dbl)  [unwired: 8 in, 1 out]
            n110 = Subtract(x=w314, y=w315) -> (x-y=w317:dbl)
            n111 = Multiply(x=w317, y=w316) -> (x*y=w313:dbl)
            n112 = Subtract(x=w315, y=w313) -> (x-y=w312:dbl)
            n113 = Add(x=w314, y=w313) -> (x+y=w311:dbl)
            n114 = Build Array(w324, w323, w321, w315, w314, w317, w312, w311) -> (w322:dbl[])
          }
          n115 = Index Array(array=w272, index (col)="Histogram\nSelected COL") -> (element=w278:dbl[])  [unwired: 1 in]
          n116 = for {
            tunnel: [w310] -> w280 mode=indexing
            tunnel: w278 -> [w310] mode=indexing
            tunnel: [w308] -> w282 mode=indexing
            i -> [w309]
            n117 = To Double Precision Float(number=w309) -> (double precision float=w308:dbl)
          }
          n118 = call <vilib>:"Histogram.vi"("intervals"=20, "X"=w278) -> ("Histogram Graph"=→"Residual's Histogram Graph":T4)  [unwired: 6 in, 3 out]
          n119 = call <vilib>:"Skewness and Kurtosis.vi"("X"=w278) -> ("kurtosis"=→"Kurtosis":dbl, "skewness"=→"Skewness":dbl)  [unwired: 8 in, 1 out]
          n120 = call "Convert to Dynamic Data"("Array"=w282) -> ("Dynamic Data Type"=w281:dynamicdata)  [unwired: 3 in]
          n121 = call "Convert to Dynamic Data2"("Array"=w280) -> ("Dynamic Data Type"=w279:dynamicdata)  [unwired: 3 in]
          n122 = Transpose 2D Array(2D array=w287) -> (transposed array=w273:dbl[][])
          "STATS Columns for each Dependent Variable's Residuals" <- w273
          n123 = call "Build XY Graph"("Y Input"=w279, "X Input"=w281) -> ("XY Graph"=→"Residual Value vs Line # XY Graph":cluster{"X":dbl[], "Y":dbl[]}[])  [unwired: 8 in, 1 out]
          n124 = Index Array(array=w267, index="Histogram\nSelected COL") -> (element=→"Residual's Variable NAME" →"Residual's Variable NAME 2":string)
          n125 = Transpose 2D Array(2D array=w273) -> (transposed array=w270:dbl[][])
          n126 = Transpose 2D Array(2D array=w272) -> (transposed array=w271:dbl[][])
          n127 = for {
            tunnel: w271 -> [w300] mode=indexing
            tunnel: w270 -> [w301] mode=indexing
            tunnel: [w295] -> w268 mode=indexing
            n128 = Index Array(array=w301, index #1=6 ("index"), index #2=7 ("index")) -> (element #1=w297:dbl, element #2=w296:dbl)
            n129 = for {
              tunnel: w300 -> [w305] mode=indexing
              tunnel: w297 -> [w307]
              tunnel: w296 -> [w304]
              tunnel: [w303] -> w295 mode=indexing
              n130 = Less?(x=w305, y=w307) -> (x < y?=w306:bool)
              n131 = Greater?(x=w305, y=w304) -> (0:w302:bool)
              n132 = Or(x=w306, y=w302) -> (x .or. y?=w303:bool)
            }
          }
          n133 = Transpose 2D Array(2D array=w268) -> (transposed array=w269:bool[][])
          "Outlier Identified (Row is Line #, Column is Variable #)" <- w269
          n134 = for {
            tunnel: w268 -> [w291] mode=indexing
            tunnel: w267 -> [w290] mode=indexing
            tunnel: [w288] -> w266 mode=indexing
            n135 = Or Array Elements(Boolean array=w291) -> (logical OR=w289:bool)
            n136 = Bundle("String"=w290, w289) -> (w288:cluster{"String":string, bool})  [unwired: 1 in]
          }
          "Column w/ OUTLIER??" <- w266
          n137 = for {
            tunnel: w269 -> [w294] mode=indexing
            tunnel: [w293] -> w264 mode=indexing
            tunnel: [w292] -> w263 mode=indexing
            n138 = Or Array Elements(Boolean array=w294) -> (logical OR=w293:bool)
            n139 = Boolean To (0,1)(Boolean=w293) -> (0, 1=w292:i16)
          }
          "Line Numbers w/ OUTLIERS" <- w264
          n140 = Array Size(array=w264) -> (size(s)=w261:i32)
          "# Datapoints in File" <- w261
          n141 = Add Array Elements(numeric array=w263) -> (sum=w262:i16)
          "# OUTLIERS" <- w262
          n142 = Divide(x=w262, y=w261) -> (x/y=w260:dbl)
          n143 = Multiply(x=w260, y=100.0) -> (x*y=→"% of Data = OUTLIER":dbl)
          "Residuals for all Dependent Variables (Value Minus Fit Value)" <- w272
        }
        frame #4 {
          # "# Points"
          # "# of Coefficients"
          # "Index by #COLS"
          n144 = Array Size(array=w329) -> (size(s)=w328:i32[])
          n145 = Index Array(array=w328, index=1) -> (element=w326:i32)
          n146 = Divide(x="Remove Coefficient\nif makes < X% Change in SSE", y=100.0) -> (x/y=w335:dbl)
          n147 = Decrement(x=w326) -> (x-1=w325:i32)
          "Full Model # of Coef." <- w325
          n148 = for {
            tunnel: w329 -> [w380] mode=indexing
            tunnel: w344 -> [w375]
            tunnel: [w376] -> w330 mode=indexing
            tunnel: w325 -> [w374]
            # "DOF"
            # "MSE"
            n149 = Reverse 1D Array(array=w380) -> (reversed array=w379:dbl[])
            n150 = Index Array(array=w379, index=0) -> (element=w377:dbl)
            n151 = Subtract(x=w375, y=w374) -> (x-y=w373:i32)
            n152 = Multiply(x=w373, y=w377) -> (x*y=w376:dbl)
          }
          "SSE Full Model(s)" <- w330
          n153 = Increment(x=w335) -> (x+1=w331:dbl)
          "SSE Ratio Must Be < THIS \nto Throw Out the Coeff." <- w331
          n154 = Transpose 2D Array(2D array=w341) -> (transposed array=w342:dbl[][])
          n155 = for {
            tunnel: w343 -> [w353]
            tunnel: w342 -> [_] mode=indexing
            tunnel: w341 -> [w358]
            shift-right: [w352] -> w339
            shift-left: dbl[][] [] -> [w351]
            tunnel: w330 -> [w350]
            tunnel: w331 -> [w348]
            shift-right: [w346] -> w333
            shift-left: bool[][] [] -> [w345]
            i -> [w357]
            # "H Matrix"
            # "Dependent\nVariables"
            # "Replace each COL in turn by 0 Array"
            # "#ROWS in H"
            n156 = Array Size(array=w358) -> (size(s)=w362:i32[])
            n157 = Index Array(array=w362, index=0) -> (element=w359:i32)
            n158 = Initialize Array(0.0 ("element"), w359) -> (w356:dbl[])
            n159 = Transpose 2D Array(2D array=w353) -> (transposed array=w355:dbl[][])
            n160 = Replace Array Subset(array=w358, new element=w356, index (col)=w357) -> (w354:dbl[][])  [unwired: 1 in]
            "Reduced Model's H Matrix" <- w354
            n161 = for {
              tunnel: w355 -> [w371] mode=indexing
              tunnel: w354 -> [w372]
              tunnel: w350 -> [w366] mode=indexing
              tunnel: [w364] -> w349 mode=indexing
              tunnel: w348 -> [w365]
              tunnel: [w363] -> w347 mode=indexing
              w370 = T8 0 items=["Least Square", "Least Absolute Residual", "Bisquare"] ("method")
              # "For all Dependent Vars."
              n162 = local read "# of Points (ROWS)"() -> (w369:i32)
              n163 = call <vilib>:"General Linear Fit.vi"("Y"=w371, "H"=w372, "method"=w370) -> ("residue"=w368:dbl)  [unwired: 7 in, 5 out]
              n164 = Multiply(x=w369, y=w368) -> (x*y=w367:dbl)
              n165 = Divide(x=w367, y=w366) -> (x/y=w364:dbl)
              n166 = Less?(x=w364, y=w365) -> (x < y?=w363:bool)
            }
            n167 = Build Array (concatenate)(w351, w349) -> (w352:dbl[][])
            n168 = Build Array (concatenate)(w345, w347) -> (w346:bool[][])
          }
          n169 = Transpose 2D Array(2D array=w339) -> (transposed array=→"F-Test----SSE Reduced Model(s) Divided by SSE Full Model = SSE Ratio":dbl[][])
          n170 = Transpose 2D Array(2D array=w333) -> (transposed array=w332:bool[][])
          "TOSS OUT Coefficients indicated by RED LED's" <- w332
        }
        frame #5 {
          # "Add DOF to last column."
          # "Generate Coefficients and MSE for the reduced models."
          n171 = case shown="True" "DO Backward Elimination\nto REDUCE # Coefficients?" {
            tunnel: w394 -> [_ w425]
            tunnel: w393 -> [_ w424]
            tunnel: [w416 w423] -> w387
            tunnel: w392 -> [_ w418]
            tunnel: w390 -> [w416 _]
            frame False {
            }
            frame True {
              # "#ROWS in H"
              # "Coeff and\nMSE in last COL"
              # "H Matrix"
              # "Dependent\nVariables"
              n172 = Array Size(array=w418) -> (size(s)=w422:i32[])
              n173 = Index Array(array=w422, index=0) -> (element=w419:i32)
              n174 = Transpose 2D Array(2D array=w425) -> (transposed array=w426:dbl[][])
              n175 = Initialize Array(0.0 ("element"), w419) -> (w417:dbl[])
              n176 = for {
                tunnel: w426 -> [w429] mode=indexing
                tunnel: w418 -> [w431]
                tunnel: [w427] -> w423 mode=indexing
                tunnel: w424 -> [w432] mode=indexing
                tunnel: w417 -> [w430]
                i -> [w428]
                # "Increments on the # of Dependent Variables"
                n177 = stacked-sequence {
                  seq-local: [w434 _ _] -> [_ w456 _]
                  seq-local: [w433 _ _] -> [_ w453 _]
                  tunnel: w432 -> [w440 w457 _]
                  tunnel: w431 -> [w439 _ _]
                  tunnel: w430 -> [w438 _ _]
                  tunnel: w429 -> [w436 _ _]
                  tunnel: [_ w452 _] -> w427
                  frame #0 {
                    w441 = T8 0 items=["Least Square", "Least Absolute Residual", "Bisquare"] ("method")
                    # "Increments on BOOLEAN  to Remove Coefficients."
                    # "Replace each COL where Indicated by TRUE with 0 Array"
                    n178 = for {
                      tunnel: w440 -> [w442] mode=indexing
                      shift-right: [w445] -> w437
                      shift-left: w439 -> [w446]
                      tunnel: w438 -> [w443]
                      i -> [w444]
                      n179 = case shown="True" w442 {
                        tunnel: w446 -> [w447 w451]
                        tunnel: [w447 w450] -> w445
                        tunnel: w444 -> [_ w449]
                        tunnel: w443 -> [_ w448]
                        frame False {
                        }
                        frame True {
                          n180 = Replace Array Subset(array=w451, new element=w448, index (col)=w449) -> (w450:dbl[][])  [unwired: 1 in]
                        }
                      }
                    }
                    "H-Matrix AFTER ZERO Value COLS ADDED" <- w437
                    n181 = call <vilib>:"General Linear Fit.vi"("Y"=w436, "H"=w437, "method"=w441) -> ("Coefficients"=w434:dbl[], "residue"=w433:dbl, "error"=→"ERROR CODE":i32)  [unwired: 7 in, 3 out]
                    "Dependent Variable MATRIX \nAssociated with H-Matrix" <- w436
                  }
                  frame #1 {
                    n182 = for {
                      tunnel: w457 -> [w462] mode=indexing
                      tunnel: w456 -> [w459] mode=indexing
                      shift-right: [w460] -> w454
                      shift-left: dbl[] [] -> [w458]
                      n183 = case shown="True" w462 {
                        tunnel: [w463 0.0] -> w461
                        tunnel: w459 -> [w463 _]
                        frame False {
                        }
                        frame True {
                        }
                      }
                      n184 = Build Array (concatenate)(w458, w461) -> (w460:dbl[])
                    }
                    n185 = Build Array (concatenate)(w454, w453) -> (w452:dbl[])
                    "Fitted Coefficients MATRIX \nAssociated with H-Matrix w/ MSE at END" <- w452
                  }
                  frame #2 {
                    n186 = Select(t=15.0, s="10 sec Pause\nSTEP to Debug?", f=0.0) -> (s? t:f=w465:dbl)
                    n187 = Multiply(x=w465, y=1000.0) -> (x*y=w470:dbl)
                    n188 = Wait Until Next ms Multiple(millisecond multiple=w470) -> ()  [unwired: 1 out]
                  }
                }
                "Dependent \nVariable INDEX" <- w428
              }
            }
          }
          n189 = Array Size(array=w387) -> (size(s)=w386:i32[])
          n190 = Index Array(array=w386, index=1) -> (element=w384:i32)
          n191 = Decrement(x=w384) -> (x-1=w382:i32)
          n192 = for {
            tunnel: w387 -> [w402] mode=indexing
            tunnel: [w406] -> w383 mode=indexing
            tunnel: w382 -> [w405]
            tunnel: [w395] -> w381
            # "95% CI on Mean"
            # "# Coef in reduced model"
            n193 = local read "# of Points (ROWS)"() -> (w407:i32)
            n194 = Reverse 1D Array(array=w402) -> (reversed array=w401:dbl[])
            n195 = for {
              N: w405 -> [_]
              tunnel: w402 -> [w411] mode=indexing
              shift-right: [w409] -> w395
              shift-left: 0 -> [w410]
              n196 = Equal To 0?(x=w411) -> (x = 0?=w412:bool)
              n197 = case shown="False" w412 {
                tunnel: w410 -> [w413 w415]
                tunnel: [w413 w414] -> w409
                frame False {
                }
                frame True {
                  n198 = Increment(x=w415) -> (x+1=w414:i32)
                }
              }
            }
            n199 = Index Array(array=w401, index=0) -> (element=w398:dbl)
            n200 = Square Root(x=w398) -> (sqrt(x)=w397:dbl)
            n201 = Subtract(x=w407, y=w395) -> (x-y=w403:i32)
            n202 = call "Students T Probability Distribution Function.vi"("degrees of freedom"=w403, "( 1 - a )"=0.95) -> ("Two-Sided"=w396:dbl)  [unwired: 9 in]
            n203 = Multiply(x=w396, y=w397) -> (x*y=w399:dbl)
            n204 = Build Array (concatenate)(w402, w403, w396, w399) -> (w406:dbl[])
          }
          "Coefficients with MSE in last Column-NUMERIC ARRAY" <- w383
          "Reduced Model \n# of Coefficients" <- w381
          n205 = Number To Exponential String(number=w383, precision (6)=i16 6) -> (E-format string=w389:string[][])  [unwired: 2 in]
        }
        frame #6 {
          # "Save the data."
          n206 = for {
            tunnel: w481 -> [w542] mode=indexing
            tunnel: w480 -> [w543]
            tunnel: w479 -> [w540] mode=indexing
            tunnel: [w537] -> w475 mode=indexing
            # "Add variable name to the first column of coefficient array."
            n207 = Index Array(array=w543, index (row)=0 ("disabled index (row)"), index (col)=w542) -> (element=w539:string)
            n208 = Insert Into Array(array=w540, index=0, new element=w539) -> (w537:string[])
          }
          n209 = Array Size(array=w475) -> (size(s)=w477:i32[])
          n210 = Index Array(array=w477, index=1) -> (element=w471:i32)
          "#COLS" <- w471
          n211 = case shown="9, Default" w471 {
            tunnel: [w482 w502 w522] -> w473
            frame 9, Default {
              n212 = Build Array("Variable_Name", "a0", "a1", "a2", "a3", "MSE", "DOF", "T-Value", "95%_CI") -> (w482:string[])
            }
            frame 15 {
              n213 = Build Array("Variable_Name", "a0", "a1", "a2", "a3", "a4", "a5", "a6", "a7", "a8", "a9", "MSE", "DOF", "T-Value", "95%_CI") -> (w502:string[])
            }
            frame 25 {
              n214 = Build Array("Variable_Name", "a0", "a1", "a2", "a3", "a4", "a5", "a6", "a7", "a8", "a9", "a10", "a11", "a12", "a13", "a14", "a15", "a16", "a17", "a18", "a19", "MSE", "DOF", "T-Value", "95%_CI") -> (w522:string[])
            }
          }
          n215 = Insert Into Array(array=w475, index (row)=0, new element=w473) -> (w472:string[][])  [unwired: 1 in]
          "Reduced Model(s) Coefficients with MSE, DOF(N-m), Student T-Value, and Model 95% CI (on Mean) in last four columns of the row" <- w472
          n216 = case shown="True" "SAVE?" {
            tunnel: w472 -> [_ w536]
            frame False {
            }
            frame True {
              n217 = call-poly <vilib>:"Write Delimited Spreadsheet.vi"("file path (dialog if empty)"="Saved Coefficient File", "2D data"=w536) -> ("error out"=→"Save Coeff error out":errorcluster)  [unwired: 12 in, 1 out]
            }
          }
        }
        frame #7 {
          w544 = TRUE ("STOPPED 2")
          "STOPPED" <- w544
          "STOPPED 2" <- w544
        }
      }
      n218 = call <vilib>:"Measures of Spread.vi"("type"=w97) -> ()  [unwired: 9 in, 2 out]
    }
  }
